vi "example sequence with cancel.vi"() -> ()   [LabVIEW 2013]
uses:
  result/result.lvclass
  standard action/wait action/wait action.lvclass
  wait without cancel/noncancellable wait.lvclass
  action/action.lvclass
  standard tokens/cancel token/cancel token.lvclass
  result/result.lvclass/result.ctl
  result/get data.vi
  result/get error.vi
  result/get generating action.vi
  result/get owning task.vi
  result/get subresults.vi
  result/get data ID.vi
  dispatcher/thread pool.lvclass
  standard reporters/event reporter/event reporter.lvclass
  standard tasks/sequence task/sequence task.lvclass
panel:
  out "data ID":string
  in  "cancel immediately?":bool
  out "cancel time":u32
  in  "cancel":bool
  out "owning task":string
  out "generating action":string
  out "error":errorcluster
  out "data":variant
  out "accessors:subresults":refnum<class "result.lvclass">[][](array[class])
  out "Array 4":string[](array[string])
  out "Array 3":string[](array[string])
  out "Array 2":errorcluster[](array[cluster])
  out "Array":variant[](array[variant])
  out "Time":u32
  out "result":refnum<class "result.lvclass">
  out "error out":errorcluster
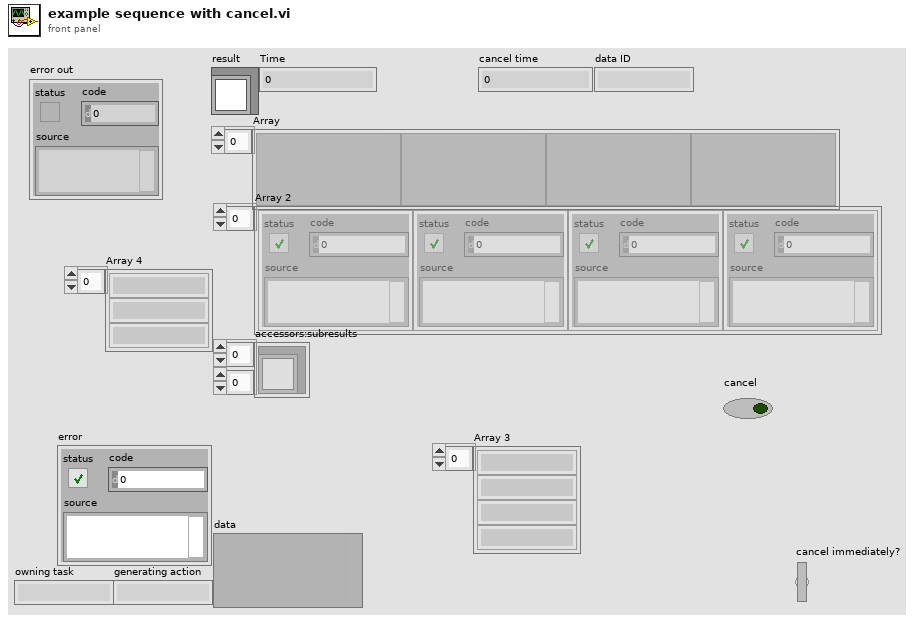
[diagram p1: front panel]
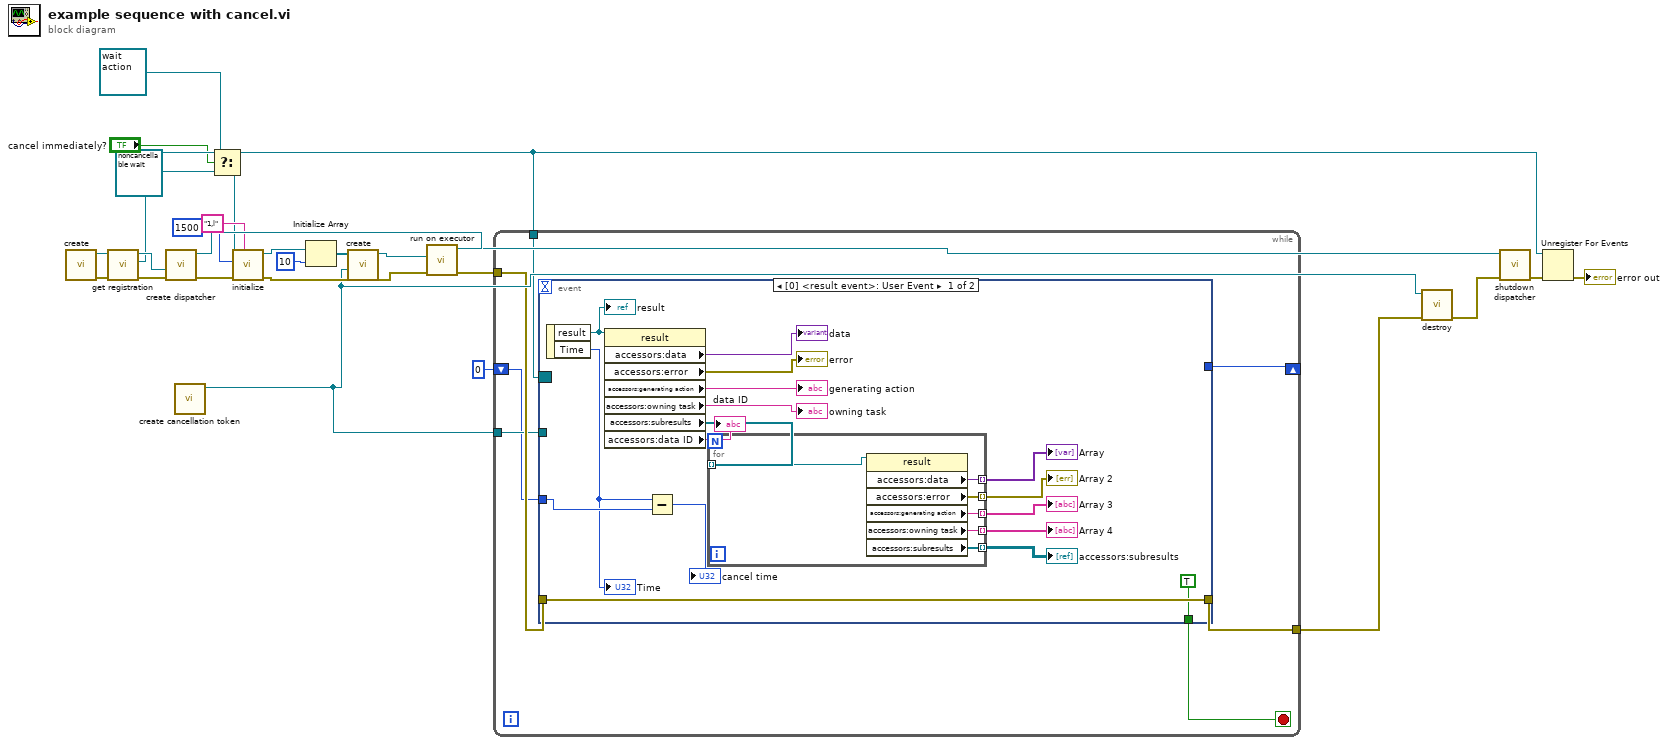
[diagram p0: block diagram]
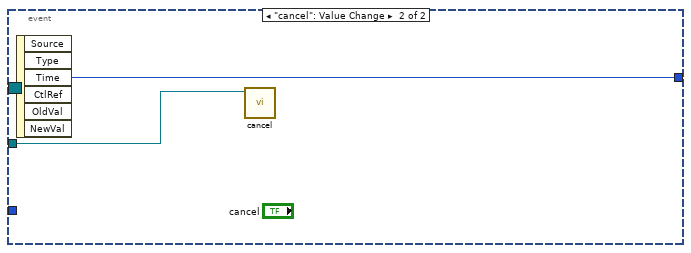
[diagram p2: hidden frame]
diagram:
  n1 = call "create.vi"() -> ("error out"=w21:errorcluster, "event reporter out"=w22:refnum<class "event reporter.lvclass">)  [unwired: 10 in]
  n2 = call "get registration.vi"("error in"=w21, "event reporter in"=w22) -> ("error out"=w19:errorcluster, "result registration"=w6:refnum<event-registration>, "event reporter out"=w20:refnum<class "event reporter.lvclass">)  [unwired: 7 in]
  n3 = call "create dispatcher.vi"("error in"=w19, "default reporter"=w20) -> ("error out"=w24:errorcluster, "dispatcher"=w26:refnum<data-value>)  [unwired: 8 in]
  n4 = call "create cancellation token.vi"() -> ("cancel token out"=w5:refnum<class "cancel token.lvclass">)  [unwired: 10 in, 1 out]
  n5 = Select(t=refnum<class "wait action.lvclass"> refnum ("wait action.lvclass"), s="cancel immediately?", f=refnum<class "noncancellable wait.lvclass"> refnum ("noncancellable wait.lvclass")) -> (s? t:f=w3:refnum<class "action.lvclass">)
  n6 = call-dynamic "initialize.vi"("action name"="1,l", "error in"=w24, "parameters"=1500, "action in"=w3) -> ("error out"=w9:errorcluster, "action out"=w13:refnum<class "action.lvclass">)  [unwired: 6 in]
  n7 = Initialize Array(w13, 10 ("dimension size")) -> (w11:refnum<class "action.lvclass">[])
  n8 = call "create.vi"("task token"=w5, "actions"=w11) -> ("sequence task out"=w10:refnum<class "sequence task.lvclass">)  [unwired: 9 in]
  n9 = call "run on executor.vi"("error in"=w9, "task"=w10, "dispatcher"=w26) -> ("error out"=w14:errorcluster, "dispatcher out"=w18:refnum<data-value>)  [unwired: 7 in]
  n10 = while {
    tunnel: w6 -> [w33]
    tunnel: [w32] -> w15
    tunnel: w14 -> [w31]
    tunnel: w5 -> [w29]
    shift-right: [w28] -> _
    shift-left: u32 0 ("Time") -> [w27]
    stop <- w30 stop-if-true
    n11 = event shown="[0] <result event>: User Event" {
      selector: w33 -> [_ _]
      dyn-events: _ -> [_ _]
      timeout: _ -> [_ _]
      tunnel: [w50 _] -> w32
      tunnel: w31 -> [w50 _]
      tunnel: [TRUE _] -> w30
      tunnel: w29 -> [_ w58]
      tunnel: [_ w57] -> w28
      tunnel: w27 -> [w37 _]
      event User Event {
        n12 = event-data() -> ("result"=w49:refnum<class "result.lvclass">, "Time"=w36:u32)  [unwired: 1 in]
        "result" <- w49
        "Time" <- w36
        n13 = property class="result"(reference=w49) -> ("accessors:data"=→"data":variant, "accessors:error"=→"error":errorcluster, "accessors:generating action"=→"generating action":string, "accessors:owning task"=→"owning task":string, "accessors:subresults"=w48:refnum<class "result.lvclass">[], "accessors:data ID"=→"data ID":string)  [unwired: 1 in, 2 out]
        n14 = Subtract(x=w36, y=w37) -> (x-y=→"cancel time":u32)
        n15 = for {
          tunnel: w48 -> [w56] mode=indexing
          tunnel: [w55] -> w47 mode=indexing
          tunnel: [w54] -> w46 mode=indexing
          tunnel: [w53] -> w45 mode=indexing
          tunnel: [w52] -> w44 mode=indexing
          tunnel: [w51] -> w43 mode=indexing
          n16 = property class="result"(reference=w56) -> ("accessors:data"=w55:variant, "accessors:error"=w54:errorcluster, "accessors:generating action"=w53:string, "accessors:owning task"=w52:string, "accessors:subresults"=w51:refnum<class "result.lvclass">[])  [unwired: 1 in, 2 out]
        }
        "Array" <- w47
        "Array 2" <- w46
        "Array 3" <- w45
        "Array 4" <- w44
        "accessors:subresults" <- w43
      }
      event "cancel": Value Change {
        n17 = event-data() -> ("Time"=w57:u32)  [unwired: 1 in, 5 out]
        n18 = call-dynamic "cancel.vi"("cancel token in"=w58) -> ()  [unwired: 9 in, 2 out]
      }
    }
  }
  n19 = call-dynamic "destroy.vi"("error in"=w15, "task token in"=w5) -> ("error out"=w7:errorcluster)  [unwired: 9 in]
  n20 = call "shutdown dispatcher.vi"("error in"=w7, "dispatcher"=w18) -> ("error out"=w17:errorcluster)  [unwired: 9 in]
  n21 = Unregister For Events(event registration refnum=w6, error in=w17) -> (error out=→"error out":errorcluster)
